vi "PID - Config (SubVI).vi"(7 "Action":enum16{"Save", "Load"}(ring)=enum."Load", 8 "error in (no error)":errorcluster, 10 "path":path, 11 "DS in":T2={"Sensor Port"=[], "Timeout"=-1, "PID"={"Output Range"={"High"=100.0, "Low"=-100.0}, "PID Tuning"={"(Kc)"=1.0, " (Ti, min)"=0.01, "(Td, min)"=0.0}, "SetPoint"=0.0}, "Machine"=0, "Invert"=FALSE, "Machine Table"=[], "Inv"={"Bool"=[], "M"=[]}} {"Machine" items=["Please Select", "Motor 1", "Motor 2", "Motor 3", "Motor 4", "Motor 5", "Motor 6", "Motor 7", "Motor 8", "Motor 9"]; "PID"."Output Range"."Low" format="%.2f"; "PID"."Output Range"."High" format="%.2f"; "PID"."PID Tuning"."(Td, min)" format="%.6f"; "PID"."PID Tuning"."(Ti, min)" format="%.6f"; "PID"."PID Tuning"."(Kc)" format="%.6f"; "Sensor Port" items=["Please Select", "LC 1", "LC 2", "LC 3", "LC 4", "LC 5", "LC 6", "LC 7", "LC 8", "TD 1", "TD 2", "TD 3", "TD 4", "TD 5", "TD 6", "TD 7", "TD 8", "TD 9", "TD 10", "TD 11", "TD 12"]}) -> (0 "error out":errorcluster, 3 "DS out":T2={"Sensor Port"=[], "Timeout"=-1, "PID"={"Output Range"={"High"=100.0, "Low"=-100.0}, "PID Tuning"={"(Kc)"=1.0, " (Ti, min)"=0.01, "(Td, min)"=0.0}, "SetPoint"=0.0}, "Machine"=0, "Invert"=FALSE, "Machine Table"=[], "Inv"={"Bool"=[], "M"=[]}} {"Machine" items=["Please Select", "Motor 1", "Motor 2", "Motor 3", "Motor 4", "Motor 5", "Motor 6", "Motor 7", "Motor 8", "Motor 9"]; "PID"."Output Range"."Low" format="%.2f"; "PID"."Output Range"."High" format="%.2f"; "PID"."PID Tuning"."(Td, min)" format="%.6f"; "PID"."PID Tuning"."(Ti, min)" format="%.6f"; "PID"."PID Tuning"."(Kc)" format="%.6f"; "Sensor Port" items=["Please Select", "LC 1", "LC 2", "LC 3", "LC 4", "LC 5", "LC 6", "LC 7", "LC 8", "TD 1", "TD 2", "TD 3", "TD 4", "TD 5", "TD 6", "TD 7", "TD 8", "TD 9", "TD 10", "TD 11", "TD 12"]})   [LabVIEW 2019]
uses:
  Controls/PID Config - Data Structure.ctl
  Controls/FGV States.ctl
  Controls/eFGV States.ctl
  Controls/Communication - LC PID.ctl
  <vilib>/Utility/config.llb/Read Key (String).vi
  <vilib>/Utility/config.llb/Write Key (String).vi
  <vilib>/Utility/config.llb/NI_LVConfig.lvlib
panel:
  out "Sensor Port":T1(ring)
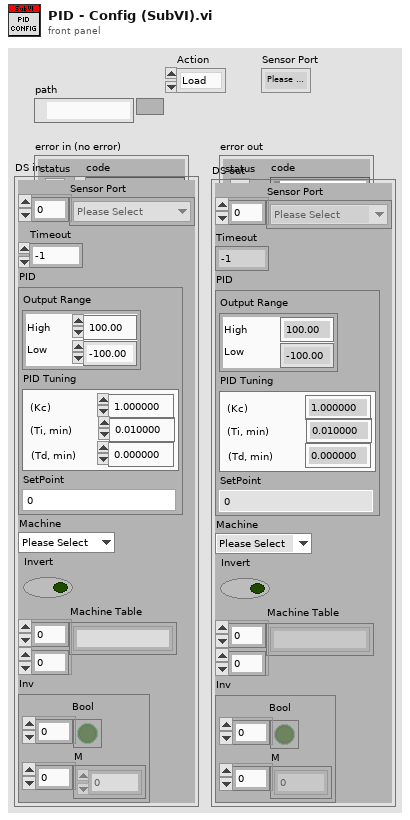
[diagram p1: front panel]
types:
  T1 = enum16{"Please Select", "LC 1", "LC 2", "LC 3", "LC 4", "LC 5", "LC 6", "LC 7", "LC 8", "TD 1", "TD 2", "TD 3", "TD 4", "TD 5", "TD 6", "TD 7", "TD 8", "TD 9", "TD 10", "TD 11", "TD 12"}
  T2 = typedef "PID Config - Data Structure.ctl" = cluster{"Sensor Port":u16[], "Timeout":i32, "PID":cluster{"Output Range":cluster{"High":dbl, "Low":dbl}, "PID Tuning":cluster{"(Kc)":dbl, " (Ti, min)":dbl, "(Td, min)":dbl}, "SetPoint":dbl}, "Machine":u16, "Invert":bool, "Machine Table":string[][], "Inv":cluster{"Bool":bool[], "M":i32[]}}
  T3 = typedef "eFGV States.ctl" = enum16{"Init", "Read", "Write", "Exit"}
  T4 = typedef "FGV States.ctl" = enum16{"Read", "Write"}
  T5 = cluster{"output range OUT":cluster{"output high":dbl, "output low":dbl}, "PID gains OUT":cluster{"proportional gain (Kc)":dbl, "integral time (Ti, min)":dbl, "derivative time (Td, min)":dbl}, "Set point":dbl}
  T6 = typedef "Communication - LC PID.ctl" = cluster{"output range":cluster{"output high":dbl, "output low":dbl}, "PID gains":cluster{"proportional gain (Kc)":dbl, "integral time (Ti, min)":dbl, "derivative time (Td, min)":dbl}, "Set point":dbl}[]
  T7 = typedef "NI_LVConfig.lvlib/Config Data RefNum.ctl" = refnum<k1>
  T8 = typedef "Communication - TD PID.ctl" = cluster{"output range OUT":cluster{"output high":dbl, "output low":dbl}, "PID gains OUT":cluster{"proportional gain (Kc)":dbl, "integral time (Ti, min)":dbl, "derivative time (Td, min)":dbl}, "Set point":dbl}[]
  T9 = cluster{"output range OUT":cluster{"output high":dbl, "output low":dbl}, "PID gains OUT":cluster{"proportional gain (Kc)":dbl, "integral time (Ti, min)":dbl, "derivative time (Td, min)":dbl}, "Set point":dbl}[]
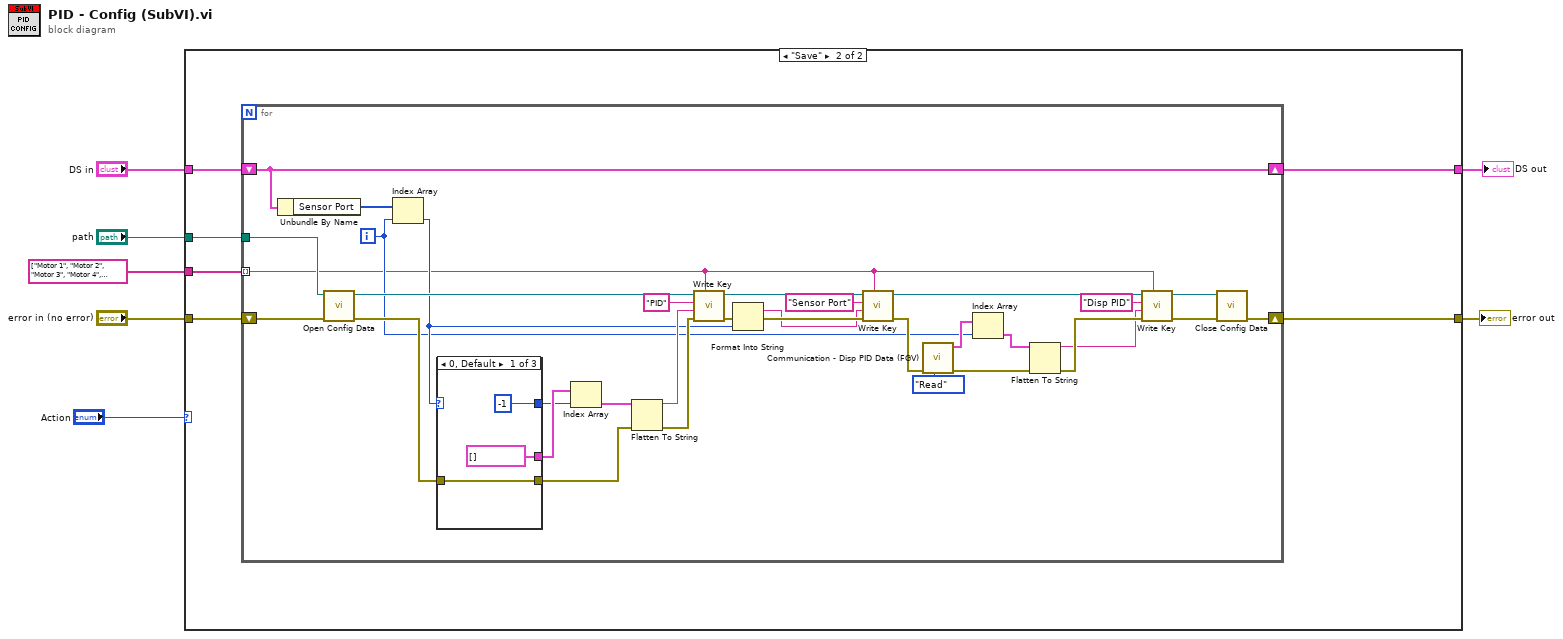
[diagram p0: block diagram]
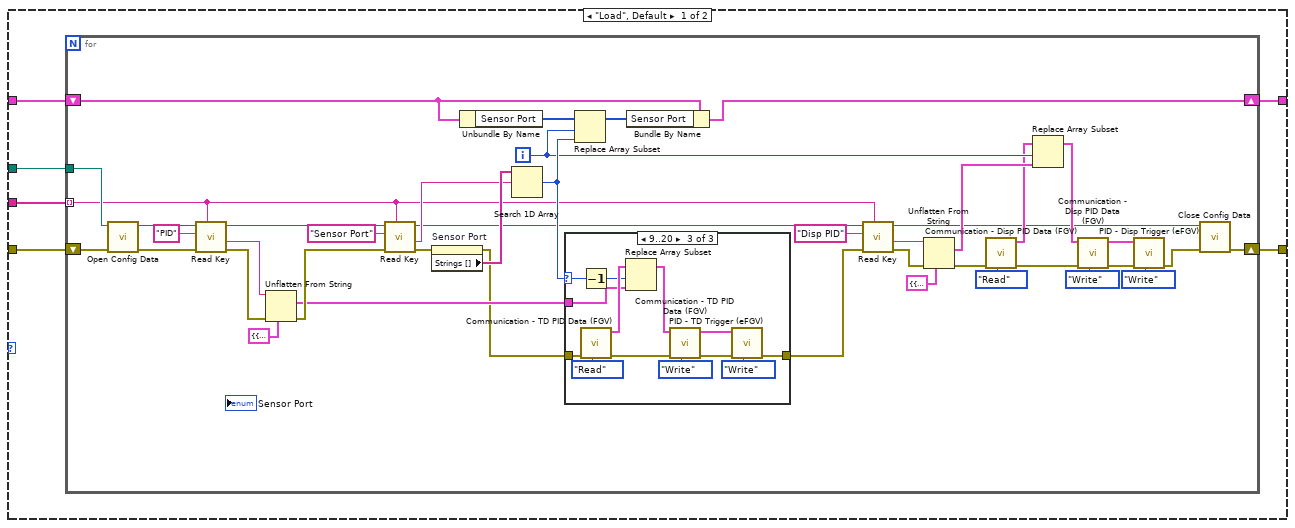
[diagram p2: hidden frame]
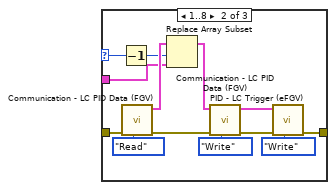
[diagram p4: hidden frame]
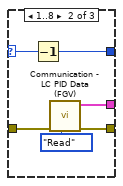
[diagram p5: hidden frame]
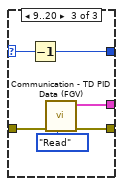
[diagram p6: hidden frame]
diagram:
  n1 = case shown="\"Save\"" "Action" {
    tunnel: "path" -> [w13 w88]
    tunnel: [w12 w87] -> w6
    tunnel: string[] ["Motor 1", "Motor 2", "Motor 3", "Motor 4", "Motor 5", "Motor 6", "Motor 7", "Motor 8", "Motor 9"] ("Strings []") -> [w11 w86]
    tunnel: "DS in" -> [w10 w85]
    tunnel: [w9 w84] -> w3
    tunnel: "error in (no error)" -> [w8 w83]
    frame "Load", Default {
      n2 = for {
        tunnel: w13 -> [w55]
        shift-right: [w15] -> w12
        shift-left: w8 -> [w53]
        tunnel: w11 -> [w31] mode=indexing
        shift-right: [w38] -> w9
        shift-left: w10 -> [w39]
        i -> [w27]
        n3 = call <vilib>:"Open Config Data.vi"("error in (no error)"=w53, "configuration file path"=w55) -> ("error out"=w49:errorcluster, "refnum"=w54:T7)  [unwired: 7 in, 1 out]
        n4 = call-poly <vilib>:"Read Key.vi"("section"=w31, "error in (no error)"=w49, "key"="PID", "refnum"=w54) -> ("error out"=w48:errorcluster, "value"=w45:string, "refnum out"=w51:T7)  [unwired: 4 in, 1 out]
        n5 = Unflatten From String(type=T5 {"output range OUT"={"output high"=0.0, "output low"=0.0}, "PID gains OUT"={"proportional gain (Kc)"=0.0, "integral time (Ti, min)"=0.0, "derivative time (Td, min)"=0.0}, "Set point"=0.0} ("element"), binary string=w45, error in (no error)=w48) -> (value=w36:T5, error out=w47:errorcluster)  [unwired: 2 in, 1 out]
        n6 = call-poly <vilib>:"Read Key.vi"("section"=w31, "error in (no error)"=w47, "key"="Sensor Port", "refnum"=w51) -> ("error out"=w43:errorcluster, "value"=w41:string, "refnum out"=w32:T7)  [unwired: 4 in, 1 out]
        n7 = property on="Sensor Port" class="Enum (strict)"(error in=w43) -> (error out=w33:errorcluster, "Strings []"=w42:string[])  [unwired: 1 in, 1 out]
        n8 = Unbundle By Name(w39) -> ("Sensor Port"=w44:u16[])
        n9 = Search 1D Array(1D array=w42, element=w41) -> (index of element=w37:i32)  [unwired: 1 in]
        n10 = case shown="9..20" w37 {
          selector: w37 -> [_ w67 w82]
          tunnel: w33 -> [w56 w68 w80]
          tunnel: [w56 w58 w71] -> w34
          tunnel: w36 -> [_ w64 w74]
          frame 0, Default {
          }
          frame 1..8 {
            n11 = Decrement(x=w67) -> (x-1=w65:i32)
            n12 = call "Communication - LC PID Data (FGV).vi"("Action"=FGV_States."Read", "error in (no error)"=w68) -> ("error out"=w62:errorcluster, "LC PID SV out"=w66:T6)  [unwired: 8 in]
            n13 = Replace Array Subset(array=w66, new element=w64, index=w65) -> (w61:T6)
            n14 = call "Communication - LC PID Data (FGV).vi"("Action"=FGV_States."Write", "error in (no error)"=w62, "LC PID SV"=w61) -> ("error out"=w59:errorcluster, "LC PID SV out"=w57:T6)  [unwired: 7 in]
            n15 = call "PID - LC Trigger (eFGV).vi"("Action"=eFGV_States."Write", "error in"=w59, "PID LC SV"=w57) -> ("error out"=w58:errorcluster)  [unwired: 6 in, 2 out]
          }
          frame 9..20 {
            n16 = Decrement(x=w82) -> (x-1=w78:i32)
            n17 = call "Communication - TD PID Data (FGV).vi"("Action"=FGV_States."Read", "error in (no error)"=w80) -> ("error out"=w76:errorcluster, "TD PID SV out"=w79:T8)  [unwired: 8 in]
            n18 = Replace Array Subset(array=w79, new element=w74, index=w78) -> (w75:T8)
            n19 = call "Communication - TD PID Data (FGV).vi"("Action"=FGV_States."Write", "error in (no error)"=w76, "TD PID SV"=w75) -> ("error out"=w72:errorcluster, "TD PID SV out"=w70:T8)  [unwired: 7 in]
            n20 = call "PID - TD Trigger (eFGV).vi"("Action"=eFGV_States."Write", "error in"=w72, "PID TD SV"=w70) -> ("error out"=w71:errorcluster)  [unwired: 6 in, 2 out]
          }
        }
        n21 = Replace Array Subset(array=w44, new element=w37, index=w27) -> (w40:u16[])
        n22 = Bundle By Name(cluster=w39, "Sensor Port"=w40) -> (w38:T2)
        n23 = call-poly <vilib>:"Read Key.vi"("section"=w31, "error in (no error)"=w34, "key"="Disp PID", "refnum"=w32) -> ("error out"=w29:errorcluster, "value"=w28:string, "refnum out"=w14:T7)  [unwired: 4 in, 1 out]
        n24 = Unflatten From String(type=T5 {"output range OUT"={"output high"=0.0, "output low"=0.0}, "PID gains OUT"={"proportional gain (Kc)"=0.0, "integral time (Ti, min)"=0.0, "derivative time (Td, min)"=0.0}, "Set point"=0.0} ("element"), binary string=w28, error in (no error)=w29) -> (value=w26:T5, error out=w24:errorcluster)  [unwired: 2 in, 1 out]
        n25 = call "Communication - Disp PID Data (FGV).vi"("Action"=FGV_States."Read", "error in (no error)"=w24) -> ("error out"=w20:errorcluster, "Disp PID SV out"=w23:T9)  [unwired: 8 in]
        n26 = Replace Array Subset(array=w23, new element=w26, index=w27) -> (w19:T9)
        n27 = call "Communication - Disp PID Data (FGV).vi"("Action"=FGV_States."Write", "error in (no error)"=w20, "Disp PID SV"=w19) -> ("error out"=w21:errorcluster, "Disp PID SV out"=w18:T9)  [unwired: 7 in]
        n28 = call "PID - Disp Trigger (eFGV).vi"("Action"=eFGV_States."Write", "error in"=w21, "PID Disp SV"=w18) -> ("error out"=w16:errorcluster)  [unwired: 6 in, 2 out]
        n29 = call <vilib>:"Close Config Data.vi"("error in (no error)"=w16, "refnum"=w14) -> ("error out"=w15:errorcluster)  [unwired: 8 in, 1 out]
      }
    }
    frame "Save" {
      n30 = for {
        tunnel: w88 -> [w121]
        shift-right: [w119] -> w87
        shift-left: w83 -> [w118]
        tunnel: w86 -> [w89] mode=indexing
        shift-right: [w117] -> w84
        shift-left: w85 -> [w117]
        i -> [w94]
        n31 = Unbundle By Name(w117) -> ("Sensor Port"=w116:u16[])
        n32 = call <vilib>:"Open Config Data.vi"("error in (no error)"=w118, "configuration file path"=w121) -> ("error out"=w115:errorcluster, "refnum"=w120:T7)  [unwired: 7 in, 1 out]
        n33 = Index Array(array=w116, index=w94) -> (element=w103:u16)
        n34 = case shown="0, Default" w103 {
          selector: w103 -> [_ w127 w136]
          tunnel: w115 -> [w123 w129 w133]
          tunnel: [w123 w128 w132] -> w110
          tunnel: [T6 [] ("LC PID SV out") w126 w131] -> w114
          tunnel: [-1 w125 w135] -> w113
          frame 0, Default {
          }
          frame 1..8 {
            n35 = Decrement(x=w127) -> (x-1=w125:u16)
            n36 = call "Communication - LC PID Data (FGV).vi"("Action"=FGV_States."Read", "error in (no error)"=w129) -> ("error out"=w128:errorcluster, "LC PID SV out"=w126:T6)  [unwired: 8 in]
          }
          frame 9..20 {
            n37 = Decrement(x=w136) -> (x-1=w135:u16)
            n38 = call "Communication - TD PID Data (FGV).vi"("Action"=FGV_States."Read", "error in (no error)"=w133) -> ("error out"=w132:errorcluster, "TD PID SV out"=w131:T8)  [unwired: 8 in]
          }
        }
        n39 = Index Array(array=w114, index=w113) -> (element=w111:T5)
        n40 = Flatten To String(anything=w111, error in (no error)=w110) -> (data string=w108:string, error out=w109:errorcluster)  [unwired: 2 in, 1 out]
        n41 = call-poly <vilib>:"Write Key.vi"("section"=w89, "error in (no error)"=w109, "value"=w108, "key"="PID", "refnum"=w120) -> ("error out"=w105:errorcluster, "refnum out"=w107:T7)  [unwired: 4 in, 1 out]
        n42 = Format Into String(error in=w105, w103) -> (resulting string=w102:string, error out=w104:errorcluster)  [unwired: 2 in]
        n43 = call-poly <vilib>:"Write Key.vi"("section"=w89, "error in (no error)"=w104, "value"=w102, "key"="Sensor Port", "refnum"=w107) -> ("error out"=w96:errorcluster, "refnum out"=w99:T7)  [unwired: 4 in, 1 out]
        n44 = call "Communication - Disp PID Data (FGV).vi"("Action"=FGV_States."Read", "error in (no error)"=w96) -> ("error out"=w93:errorcluster, "Disp PID SV out"=w95:T9)  [unwired: 8 in]
        n45 = Index Array(array=w95, index=w94) -> (element=w91:T5)
        n46 = Flatten To String(anything=w91, error in (no error)=w93) -> (data string=w90:string, error out=w92:errorcluster)  [unwired: 2 in, 1 out]
        n47 = call-poly <vilib>:"Write Key.vi"("section"=w89, "error in (no error)"=w92, "value"=w90, "key"="Disp PID", "refnum"=w99) -> ("error out"=w100:errorcluster, "refnum out"=w98:T7)  [unwired: 4 in, 1 out]
        n48 = call <vilib>:"Close Config Data.vi"("error in (no error)"=w100, "refnum"=w98) -> ("error out"=w119:errorcluster)  [unwired: 8 in, 1 out]
      }
    }
  }
  "error out" <- w6
  "DS out" <- w3
